vi "Get Map Collection Data Size.vi"(8 "error in (no error)":errorcluster, 10 "Data String":u8[](array[numeric]), 11 "Type Descriptor":i16[](array[numeric])) -> (0 "error out":errorcluster, 2 "Data Size":i32)   [LabVIEW 2017, in "Composition.lvlib"]
doc: "Gets the data size of a map collection."
uses:
  Composition.lvlib
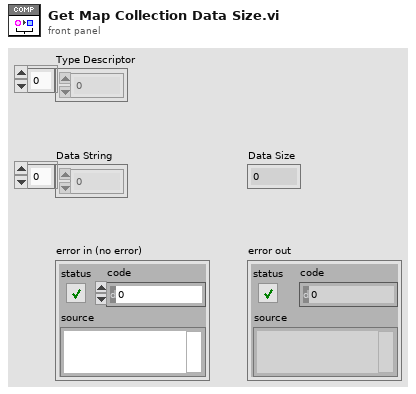
[diagram p1: front panel]
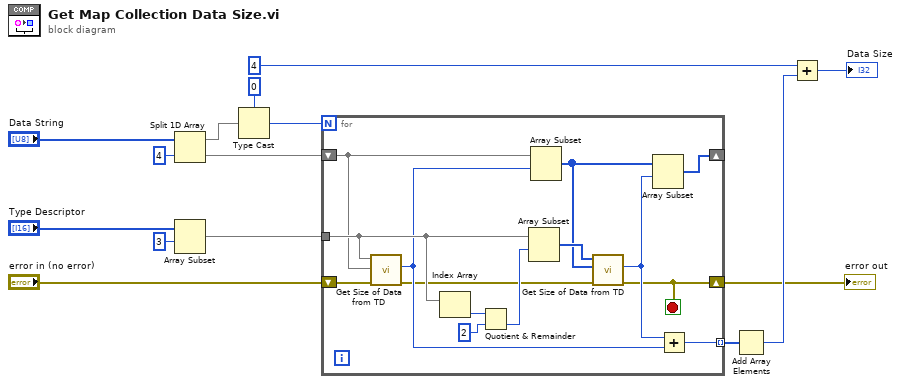
[diagram p0: block diagram]
diagram:
  n1 = Split 1D Array(array="Data String", index=4) -> (first subarray=w12:u8[], second subarray=w10:u8[])
  n2 = Array Subset(array="Type Descriptor", index=3) -> (w11:i16[])  [unwired: 1 in]
  n3 = Type Cast(type=0, x=w12) -> (*(type *) &x=w8:i32)
  n4 = for {
    N: w8 -> [_]
    tunnel: w11 -> [w29]
    shift-right: [w22] -> _
    shift-left: w10 -> [w27]
    tunnel: [w19] -> w7 mode=indexing
    shift-right: [w16] -> w2
    shift-left: "error in (no error)" -> [w18]
    stop <- w16 stop-if-true
    n5 = call "Get Size of Data from TD.vi"("error in (no error)"=w18, "Data String"=w27, "Type Descriptor"=w29) -> ("error out"=w17:errorcluster, "Size of Data"=w20:i32)  [unwired: 7 in]
    n6 = Index Array(array=w29) -> (element=w25:i16)  [unwired: 1 in]
    n7 = Quotient & Remainder(x=w25, y=i16 2) -> (floor(x/y)=w24:i16)  [unwired: 1 out]
    n8 = Array Subset(array=w29, index=w24) -> (w28:i16[])  [unwired: 1 in]
    n9 = Array Subset(array=w27, index=w20) -> (w23:u8[])  [unwired: 1 in]
    n10 = call "Get Size of Data from TD.vi"("error in (no error)"=w17, "Data String"=w23, "Type Descriptor"=w28) -> ("error out"=w16:errorcluster, "Size of Data"=w21:i32)  [unwired: 7 in]
    n11 = Array Subset(array=w23, index=w21) -> (w22:u8[])  [unwired: 1 in]
    n12 = Add(x=w21, y=w20) -> (x+y=w19:i32)
  }
  "error out" <- w2
  n13 = Add Array Elements(numeric array=w7) -> (sum=w6:i32)
  n14 = Add(x=4 ("value"), y=w6) -> (x+y=→"Data Size":i32)
